vi "Enqueue Message (Array).vi"(6 "Priority Message? Array":bool[](array[boolean]) caption="우선순위 메시지? 배열", 8 "error in (no error)":errorcluster caption="에러 입력(에러 없음)", 9 "Message Data Array":variant[](array[variant]) caption="메시지 데이터 배열", 10 "Message Array":string[](array[string]) caption="메시지 배열", 11 "Message Queue":refnum<queue> caption="메시지 큐") -> (0 "error out":errorcluster caption="에러 출력", 3 "dup Message Queue":refnum<queue> caption="메시지 큐 복제")   [LabVIEW 2018, in "Message Queue.lvlib"]
doc: "일반 메시지의 경우, 메시지를 큐에 추가합니다. 우선순위 메시지의 경우, 메시지를 큐의 앞쪽에 추가합니다."
uses:
  Message Queue.lvlib
  Message Cluster.ctl
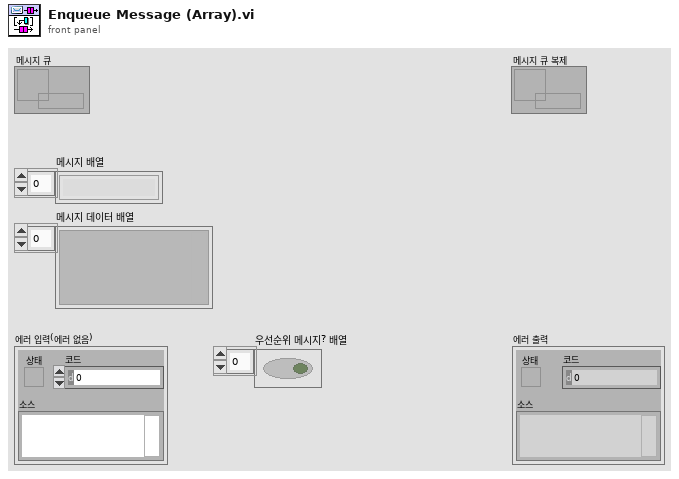
[diagram p1: front panel]
types:
  T1 = typedef "Message Queue.lvlib/Message Cluster.ctl" = cluster{"Message":string, "Message Data":variant}
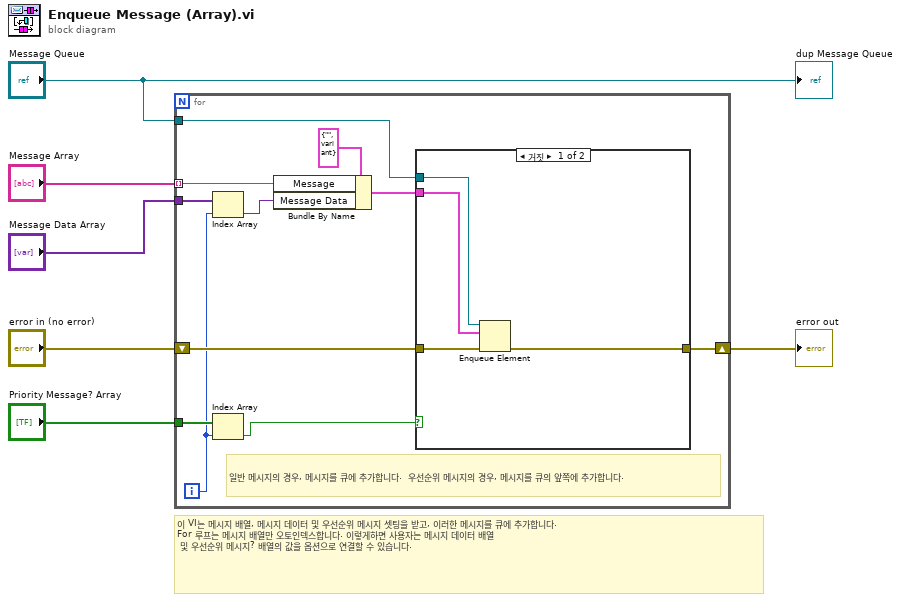
[diagram p0: block diagram]
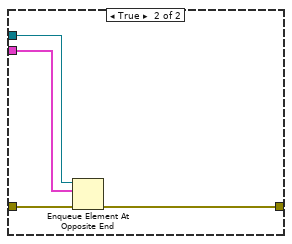
[diagram p2: hidden frame]
diagram:
  # "이 VI는 메시지 배열, 메시지 데이터 및 우선순위 메시지 셋팅을 받고, 이러한 메시지를 큐에 추가합니다.\nFor 루프는 메시지 배열만 오토인덱스합니다. 이렇게하면 사용자는 메시지 데이터 배열\n 및 우선순위 메시지? 배열의 값을 옵션으로 연결할 수 있습니다."
  n1 = for {
    tunnel: "Message Queue" -> [w14]
    tunnel: "Message Array" -> [w12] mode=indexing
    tunnel: "Message Data Array" -> [w11]
    tunnel: "Priority Message? Array" -> [w9]
    shift-right: [w15] -> w5
    shift-left: "error in (no error)" -> [w16]
    i -> [w7]
    # "일반 메시지의 경우, 메시지를 큐에 추가합니다.  우선순위 메시지의 경우, 메시지를 큐의 앞쪽에 추가합니다."
    n2 = Index Array(array=w11, index=w7) -> (element=w10:variant)
    n3 = Index Array(array=w9, index=w7) -> (element=w8:bool)
    n4 = Bundle By Name(cluster=T1 {"Message"="", "Message Data"=variant} ("Message Cluster"), "Message"=w12, "Message Data"=w10) -> (w13:T1)
    n5 = case shown="거짓" w8 {
      tunnel: w16 -> [w21 w25]
      tunnel: [w20 w24] -> w15
      tunnel: w14 -> [w19 w23]
      tunnel: w13 -> [w18 w22]
      frame False {
        n6 = Enqueue Element(queue=w19, element=w18, error in (no error)=w21) -> (error out=w20:errorcluster)  [unwired: 1 in, 2 out]
      }
      frame True {
        n7 = Enqueue Element At Opposite End(queue=w23, element=w22, error in (no error)=w25) -> (error out=w24:errorcluster)  [unwired: 1 in, 2 out]
      }
    }
  }
  "error out" <- w5
  "dup Message Queue" <- "Message Queue"
